vi "Lookup Constant.vi"(8 "error in (no error)":errorcluster, 10 "Constant Name":string, 11 "Sequence Constants in":refnum<class "Sequence Constants.lvclass">) -> (0 "error out":errorcluster, 2 "Element":refnum<class "Config Element.lvclass">, 3 "Sequence Constants out":refnum<class "Sequence Constants.lvclass">)   [LabVIEW 2020, in "VolatusSeqConfig.lvlib" / "Sequence Constants.lvclass"]
uses:
  Sequence Constants.lvclass
  lv-cdm/CDM-Config/Config Element/Config Element.lvclass
  Sequence Constants.lvclass/Sequence Constants.ctl
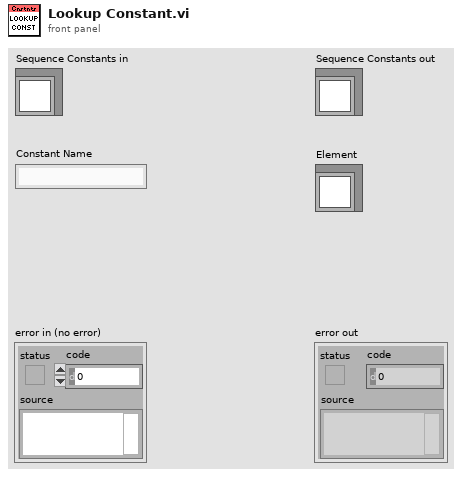
[diagram p1: front panel]
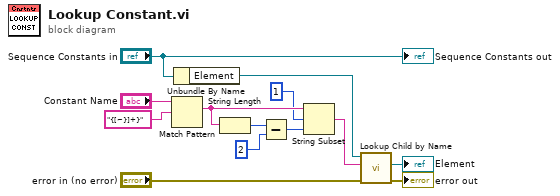
[diagram p0: block diagram]
diagram:
  n1 = Match Pattern(string="Constant Name", regular expression="{[~}]+}") -> (match substring=w4:string)  [unwired: 1 in, 3 out]
  n2 = Unbundle By Name("Sequence Constants in") -> ("Element"=w12:refnum<class "Config Element.lvclass">)
  n3 = String Length(string=w4) -> (length=w6:i32)
  n4 = Subtract(x=w6, y=2) -> (x-y=w3:i32)
  n5 = String Subset(string=w4, offset (0)=1, length (rest)=w3) -> (substring=w1:string)
  n6 = call "Lookup Child by Name.vi"("error in (no error)"="error in (no error)", "Name"=w1, "Config Element in"=w12) -> ("error out"=→"error out":errorcluster, "Child"=→"Element":refnum<class "Config Element.lvclass">)  [unwired: 5 in, 2 out]
  "Sequence Constants out" <- "Sequence Constants in"
